vi "enum+num_to_string.vi"(1 "Numeric":dbl, 2 "SCIPI":T1 items=["*IDN?", "*SAV 1", "*RCL 1", "INSTTrument CH1", "INSTTrument CH2", "INSTrument?", "MEASure:CURRent? CH1", "MEASure:CURRent? CH2", "MEASure:VOLTage? CH1", "MEASure:VOLTage? CH2", "MEASure:POWEr? CH1", "MEASure:POWEr? CH2", "CH1:CURRent?", "CH2:CURRent?", "CH1:VOLTage? ", "CH2:VOLTage? ", "OUTPut CH1,ON", "OUTPut CH1,OFF", "OUTPut CH2,ON", "OUTPut CH2,OFF", "OUTPut CH3,ON", "OUTPut CH3,OFF", "OUTPut:TRACK 0", "OUTPut:TRACK 1", "OUTPut:TRACK 2", "OUTPut:WAVE CH1,ON", "OUTPut:WAVE CH1,OFF", "OUTPut:WAVE CH2,ON", "OUTPut:WAVE CH2,OFF"]) -> (0 "concatenated string":string)   [LabVIEW 2020]
uses:
  controls/SCPI_enum.ctl
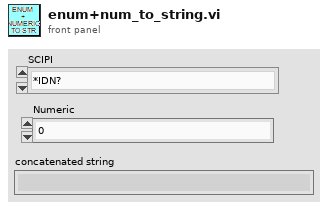
[diagram p1: front panel]
types:
  T1 = typedef "SCPI_enum.ctl" = u16
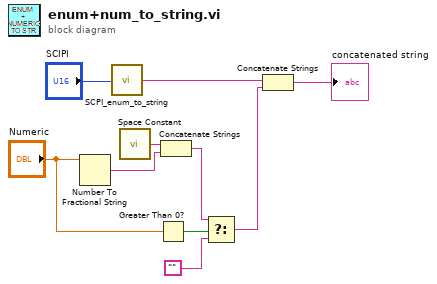
[diagram p0: block diagram]
diagram:
  n1 = Number To Fractional String(number="Numeric") -> (F-format string=w7:string)  [unwired: 3 in]
  n2 = call "SCPI_enum_to_string.vi"("SCPI"="SCIPI") -> ("resulting string 2"=w8:string)
  n3 = call <vilib>:"Space Constant.vi"() -> ("String"=w10:string)
  n4 = Greater Than 0?(x="Numeric") -> (x > 0?=w5:bool)
  n5 = Concatenate Strings(w10, w7) -> (w4:string)
  n6 = Select(t=w4, s=w5, f="") -> (s? t:f=w3:string)
  n7 = Concatenate Strings(w8, w3) -> (→"concatenated string":string)
